vi "download id.vi"(8 "error in (no error)":errorcluster, 10 "id":i16, 11 "TCP in":refnum<k5>) -> (0 "error out":errorcluster, 3 "TCP out":refnum<k5>)   [LabVIEW 2020]
panel:
  out "B/sec":dbl format="%#.4p"
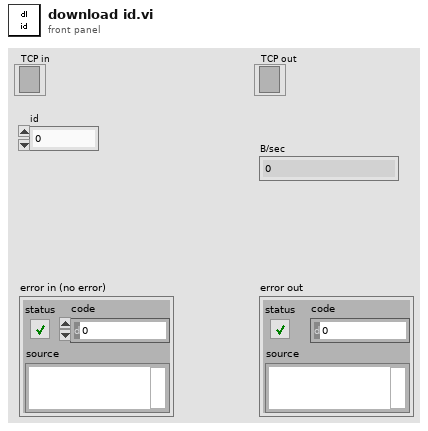
[diagram p1: front panel]
types:
  T1 = enum16{"open", "replace", "create", "open or create", "replace or create", "replace or create with confirmation"}
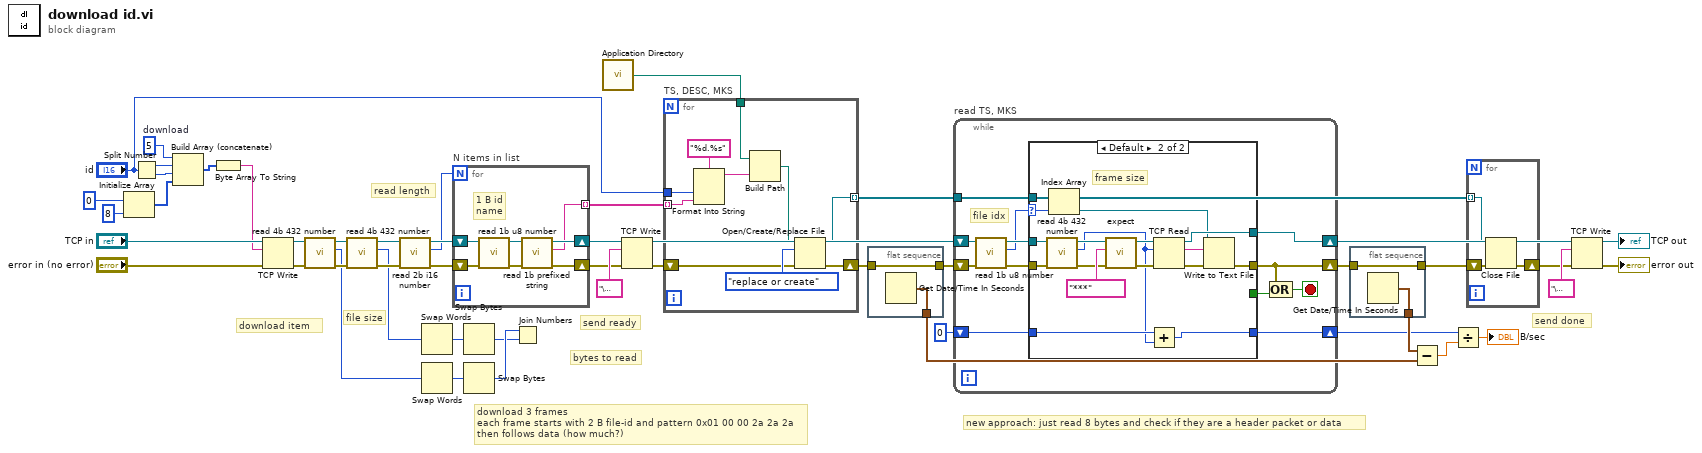
[diagram p0: block diagram]
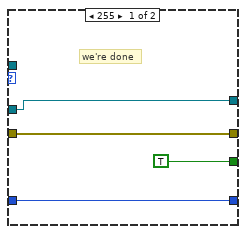
[diagram p2: hidden frame]
diagram:
  w43 = u8 5  # download
  # "send done"
  # "bytes to read"
  # "new approach: just read 8 bytes and check if they are a header packet or data"
  # "download 3 frames\neach frame starts with 2 B file-id and pattern 0x01 00 00 2a 2a 2a\nthen follows data (how much?)"
  # "file size"
  # "send ready"
  # "read length"
  # "download item"
  n1 = Initialize Array(u8 0, 8 ("dimension size")) -> (w25:u8[])
  n2 = Split Number(x="id") -> (hi(x)=w40:u8, lo(x)=w26:u8)
  n3 = Build Array (concatenate)(w43, w40, w26, w25) -> (w42:u8[])
  n4 = Byte Array To String(unsigned byte array=w42) -> (string=w41:string)
  n5 = TCP Write(connection ID="TCP in", data in=w41, error in (no error)="error in (no error)") -> (connection ID out=w17:refnum<k5>, error out=w16:errorcluster)  [unwired: 1 in, 1 out]
  n6 = call "read 4b 432 number.vi"("error in (no error)"=w16, "TCP Network Connection in"=w17) -> ("error out"=w39:errorcluster, "number"=w21:u32, "TCP Network Connection out"=w38:refnum<k5>)  [unwired: 7 in]
  n7 = call "read 4b 432 number.vi"("error in (no error)"=w39, "TCP Network Connection in"=w38) -> ("error out"=w37:errorcluster, "number"=w32:u32, "TCP Network Connection out"=w36:refnum<k5>)  [unwired: 7 in]
  n8 = call "read 2b i16 number.vi"("error in (no error)"=w37, "TCP Network Connection in"=w36) -> ("error out"=w34:errorcluster, "number"=w33:i16, "TCP Network Connection out"=w35:refnum<k5>)  [unwired: 7 in]
  n9 = Swap Words(1:w32) -> (0:w24:u32)
  n10 = Swap Words(1:w21) -> (0:w22:u32)
  n11 = for "N items in list" {
    N: w33 -> [_]
    shift-right: [w52] -> w44
    shift-left: w35 -> [w56]
    shift-right: [w51] -> w45
    shift-left: w34 -> [w55]
    tunnel: [w50] -> w29 mode=indexing
    # "1 B id\nname"
    n12 = call "read 1b u8 number.vi"("error in (no error)"=w55, "TCP Network Connection in"=w56) -> ("error out"=w54:errorcluster, "TCP Network Connection out"=w53:refnum<k5>)  [unwired: 7 in, 1 out]
    n13 = call "read 1b prefixed string.vi"("error in (no error)"=w54, "TCP Network Connection in"=w53) -> ("error out"=w51:errorcluster, "data out"=w50:string, "TCP Network Connection out"=w52:refnum<k5>)  [unwired: 7 in]
  }
  n14 = Swap Bytes(anything=w24) -> (byte swapped=w18:u32)
  n15 = Swap Bytes(anything=w22) -> (byte swapped=w19:u32)
  n16 = Join Numbers(hi=w19, lo=w18) -> ()  [unwired: 1 out]
  n17 = call <vilib>:"Application Directory.vi"() -> ("Application Directory"=w30:path)
  n18 = TCP Write(connection ID=w44, data in="\u0001", error in (no error)=w45) -> (connection ID out=w23:refnum<k5>, error out=w46:errorcluster)  [unwired: 1 in, 1 out]
  n19 = for "TS, DESC, MKS" {
    shift-right: [w57] -> w8
    shift-left: w46 -> [w59]
    tunnel: "id" -> [w65]
    tunnel: w30 -> [w63]
    tunnel: w29 -> [w62] mode=indexing
    tunnel: [w58] -> w20 mode=indexing
    n20 = Format Into String(format string="%d.%s", w65, w62) -> (resulting string=w64:string)  [unwired: 2 in, 1 out]
    n21 = Build Path(base path=w63, name or relative path=w64) -> (appended path=w61:path)
    n22 = Open/Create/Replace File(file path (use dialog)=w61, error in=w59, operation (0:open)=T1."replace or create") -> (refnum out=w58:refnum<file>, error out=w57:errorcluster)  [unwired: 3 in, 1 out]
  }
  n23 = flat-sequence {
    tunnel: [w68] -> w9
    tunnel: w8 -> [w68]
    tunnel: [w67] -> w4
    frame #0 {
      n24 = Get Date/Time In Seconds() -> (seconds since 1Jan1904=w67:timestamp)
    }
  }
  n25 = while "read TS, MKS" {
    shift-right: [w75] -> w7
    shift-left: w9 -> [w80]
    shift-right: [w79] -> w12
    shift-left: w23 -> [w76]
    tunnel: w20 -> [w73]
    shift-right: [w70] -> w3
    shift-left: u64 0 -> [w69]
    stop <- w78 stop-if-true
    # "file idx"
    n26 = call "read 1b u8 number.vi"("error in (no error)"=w80, "TCP Network Connection in"=w76) -> ("error out"=w77:errorcluster, "number"=w72:u8, "TCP Network Connection out"=w74:refnum<k5>)  [unwired: 7 in]
    n27 = case shown="Default" w72 {
      selector: w72 -> [_ w89]
      tunnel: [w84 w101] -> w79
      tunnel: w77 -> [w83 w99]
      tunnel: [w83 w94] -> w75
      tunnel: w74 -> [w84 w92]
      tunnel: w73 -> [_ w90]
      tunnel: [TRUE _] -> w71
      tunnel: [w81 w86] -> w70
      tunnel: w69 -> [w81 w87]
      frame 255 {
        # "we're done"
      }
      frame Default {
        # "frame size"
        n28 = call "read 4b 432 number.vi"("error in (no error)"=w99, "TCP Network Connection in"=w92) -> ("error out"=w93:errorcluster, "number"=w85:u32, "TCP Network Connection out"=w91:refnum<k5>)  [unwired: 7 in]
        n29 = Index Array(array=w90, index=w89) -> (element=w88:refnum<file>)
        n30 = call "expect.vi"("error in (no error)"=w93, "data expected"="***" ("data in"), "TCP Network Connection in"=w91) -> ("error out"=w98:errorcluster, "TCP Network Connection out"=w97:refnum<k5>)  [unwired: 6 in, 1 out]
        n31 = Add(x=w87, y=w85) -> (x+y=w86:u64)
        n32 = TCP Read(connection ID=w97, bytes to read=w85, error in (no error)=w98) -> (connection ID out=w101:refnum<k5>, data out=w95:string, error out=w100:errorcluster)  [unwired: 2 in]
        n33 = Write to Text File(file (use dialog)=w88, text=w95, error in=w100) -> (error out=w94:errorcluster)  [unwired: 1 in, 2 out]
      }
    }
    n34 = Compound Arithmetic op=OR(w75, w71) -> (w78:bool)
  }
  n35 = flat-sequence {
    tunnel: [w103] -> w6
    tunnel: w7 -> [w103]
    tunnel: [w102] -> w5
    frame #0 {
      n36 = Get Date/Time In Seconds() -> (seconds since 1Jan1904=w102:timestamp)
    }
  }
  n37 = Subtract(x=w5, y=w4) -> (x-y=w2:dbl)
  n38 = Divide(x=w3, y=w2) -> (x/y=→"B/sec":dbl)
  n39 = for {
    shift-right: [w106] -> w14
    shift-left: w6 -> [w105]
    tunnel: w20 -> [w104] mode=indexing
    n40 = Close File(refnum=w104, error in=w105) -> (error out=w106:errorcluster)  [unwired: 1 out]
  }
  n41 = TCP Write(connection ID=w12, data in="\u0001", error in (no error)=w14) -> (connection ID out=→"TCP out":refnum<k5>, error out=→"error out":errorcluster)  [unwired: 1 in, 1 out]
